vi "Get host time.vi"() -> (0 "TU current time":timestamp, 1 "BR current time":timestamp, 2 "TU time":dbl format="%#.10f", 3 "BR time":dbl format="%#.10f")   [LabVIEW 2018]
panel:
  out "current time":timestamp
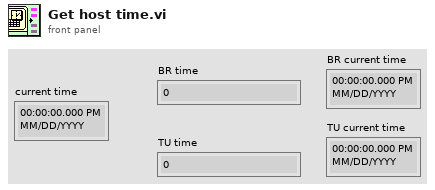
[diagram p1: front panel]
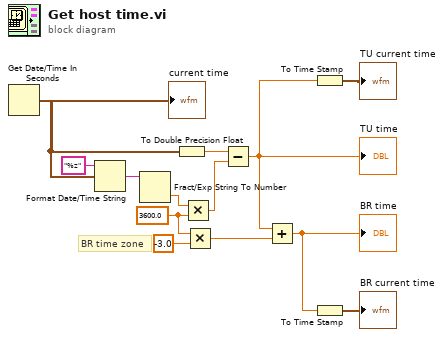
[diagram p0: block diagram]
diagram:
  w7 = 3600.0 ("y")
  # "BR time zone"
  n1 = Get Date/Time In Seconds() -> (seconds since 1Jan1904=w12:timestamp)
  "current time" <- w12
  n2 = Format Date/Time String(time format string (%c)="%z", seconds (now)=w12) -> (date/time string=w10:string)  [unwired: 1 in]
  n3 = Fract/Exp String To Number(string=w10) -> (number=w9:dbl)  [unwired: 3 in, 1 out]
  n4 = To Double Precision Float(number=w12) -> (double precision float=w13:dbl)
  n5 = Multiply(x=w9, y=w7) -> (x*y=w8:dbl)
  n6 = Multiply(x=w7, y=-3.0) -> (x*y=w5:dbl)
  n7 = Subtract(x=w13, y=w8) -> (x-y=w4:dbl)
  "TU time" <- w4
  n8 = Add(x=w4, y=w5) -> (x+y=w3:dbl)
  "BR time" <- w3
  n9 = To Time Stamp(1:w4) -> (0:→"TU current time":timestamp)
  n10 = To Time Stamp(1:w3) -> (0:→"BR current time":timestamp)
